vi "editDialog.vi"(0 "reference":refnum<class "StateNode.lvclass">, 1 "insidePackageNode":bool, 5 "error in (no error)":errorcluster) -> (14 "reference out":refnum<class "StateNode.lvclass">, 15 "changeConnection":T1, 16 "cancel":bool, 19 "error out":errorcluster)   [LabVIEW 2012, in "StateNode.lvclass"]
doc: "Edit Dialog"
uses:
  <resource>/Framework/Providers/Open_GDS/UML/StateNode_class/StateNode.lvclass
  <resource>/Framework/Providers/Open_GDS/UML/AbstractNode_class/private/NodeConnectionStatsType.ctl
  <resource>/Framework/Providers/Open_GDS/UML/ContextHelp/ContextHelp_HelpTexts.ctl
  <resource>/Framework/Providers/Open_GDS/UML/MultiLineString_class/MultiLineString.lvclass
  <resource>/Framework/Providers/Open_GDS/UML/AbstractNode_class/AbstractNode.lvclass
panel:
  in  "Action":string
  in  "OK Button":bool
  in  "Cancel Button":bool
  in  "Help":bool
  in  "State":string
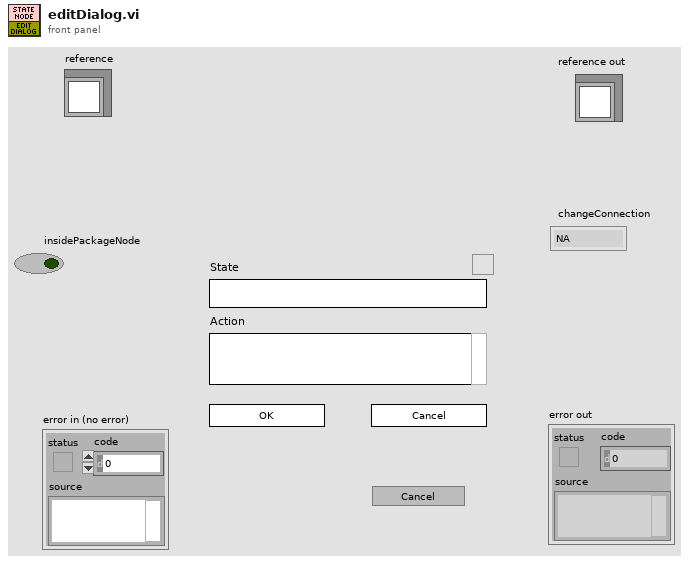
[diagram p1: front panel]
types:
  T1 = typedef "AbstractNode.lvclass/NodeConnectionStatsType.ctl" = enum16{"NA", "Connect", "DisConnect"}
  T2 = typedef "ContextHelp_HelpTexts.ctl" = enum16{"None(Hide)", "Default", "Help", "Welcome", "GettingStarted", "ClassDiagram_Help", "SequenceDiagram_Help", "UseCaseDiagram_Help", "BSelect", "BClass", "BInterface", "BPackage", "BNote", "BDependency", "BInheritance", "BInterfaceImplementation", "BAssociation", "BAggregation", "BCompAggregation", "BNoteConnector", "BObject", "BActionBar", "BCall", "BSystem", "BActor", "BUseCase", "BGeneralization", "BIncludes", "BExtends", "BUseCaseDiagramAssociation", "ClassRelationshipEdge editDialog_Bent Style", "ClassRelationshipEdge editDialog_RelationType", "ClassRelationshipEdge editDialog_Reverse association", "ClassRelationshipEdge editDialog_Start label", "ClassRelationshipEdge editDialog_Middle label", "ClassRelationshipEdge editDialog_End label", "UMLEditor reversedEngineering_Pathes", "ReversedEngineering StateReverseDialog_Help", "ReversedEngineering StateQueuedSettings_Help", "UMLEditor reversedEngineering_AddTopVIs", "UMLEditor reversedEngineering_AddClasses", "UMLEditor reversedEngineering_AddDirs", "UMLEditor reversedEngineering_Recursively", "UMLEditor reversedEngineering_Remove", "UMLEditor reversedEngineering_ClearList", "UMLEditor reversedEngineering_HideSubAss", "UMLEditor reversedEngineering_CreateTypes", "UMLEditor reversedEngineering_OnlyInheritance", "UMLEditor reversedEngineering_CreateApplication", "UMLEditor reversedEngineering_OK", "UMLEditor reversedEngineering_Cancel", "UMLEditor reversedEngineering_Help", "UMLEditor createWizardScriptFile_ScriptfilePath", "UMLEditor createWizardScriptFile_ClassPath", "UMLEditor createWizardScriptFile_Use", "UMLEditor createWizardScriptFile_PrivateDirName", "UMLEditor createWizardScriptFile_DirAppend", "UMLEditor createWizardScriptFile_Separator Character", "UMLEditor createWizardScriptFile_OK", "UMLEditor createWizardScriptFile_Cancel", "UMLEditor createWizardScriptFile_Help", "ClassNode editDialog_Class Name", "InterfaceNode editDialog_Class Name", "ClassNode editDialog_Attribute", "ClassNode editDialog_Methods", "InterfaceNode editDialog_Methods", "ClassNode editDialog_connection", "InterfaceNode editDialog_connection", "ClassNode editDialog_StereoType", "ClassNode editDialog_ShowAttrib", "ClassNode editDialog_ShowMethods", "ClassNode editDialog_ClassPath", "ClassNode editDialog_AddAttribute", "ClassNode editDialog_AddMethod", "InterfaceNode editDialog_AddMethod", "ClassNode AttributeGuide_AttributeName", "ClassNode AttributeGuide_Array?", "ClassNode AttributeGuide_Data Type", "ClassNode AttributeGuide_RefName", "ClassNode AttributeGuide_Preview", "ClassNode AttributeGuide_OK", "ClassNode AttributeGuide_Cancel", "ClassNode MethodGuide_Visibility", "ClassNode MethodGuide_Method Name", "ClassNode MethodGuide_Preview", "ClassNode MethodGuide_OK", "ClassNode MethodGuide_Cancel", "CallNode EditCallProperties_AllButtons", "ObjectNode EditObjectlProperties_AllButtons", "ActorNode EditActorProperties_AllButtons", "UseCaseRelationshipNode EditUseCaselProperties_AllButtons", "UseCaseNode EditUseCaselProperties_AllButtons", "SystemNode EditSystemProperties_AllButtons", "ReversedEngineering UpdateAttributes_AllButtons", "StateNode editDialog_AllButtons", "StateTransition editDialog_AllButtons", "ArrangeNodes Main_Picture", "ArrangeNodes Main_Zoom", "ArrangeNodes Main_Auto Zoom", "ArrangeNodes Main_shorten", "ArrangeNodes Main_Min Length", "ArrangeNodes Main_Max Length", "ArrangeNodes Main_increase", "ArrangeNodes Main_decrease", "ArrangeNodes Main_Shake", "ArrangeNodes Main", "BState", "BInitialState", "BFinalState", "BStateTransition", "StateDiagram_Help", "StateDiagram_PropertiesAllButtons", "ReversedEngineering StateReverseDialog_ClearStates", "ReversedEngineering StateReverseDialog_UseQueuedStateMachines", "ReversedEngineering StateReverseDialog_QueuedSettings", "ReversedEngineering StateReverseDialog_SearchForVIs", "ReversedEngineering StateReverseDialog_SearchCriteria", "OptionsDialog_ClassBasePath", "OptionsDialog_VIPath", "OptionsDialog_ApplicationPath", "OptionsDialog_WizDir", "OptionsDialog_IniFilePath", "OptionsDialog_DefineColors", "OptionsDialog_Help", "OptionsDialog_CreateTypes", "ClassRelationshipEdge editDialog_SplitWire"}
  T3 = typedef "StateNode.lvclass/ObjectAttributes.ctl" = cluster{"Base class":T4, "state":refnum<class "MultiLineString.lvclass">, "action":refnum<class "MultiLineString.lvclass">, "DEFAULT_WIDTH":i32, "DEFAULT_HEIGHT":i32}
  T4 = typedef "RectangularNode.lvclass/ObjectAttributes.ctl" = cluster{"Base class":T5, "bounds":T6}
  T5 = typedef "AbstractNode.lvclass/ObjectAttributes.ctl" = cluster{"parent":refnum<class "AbstractNode.lvclass">, "children":refnum<class "AbstractNode.lvclass">[], "Hidden":bool}
  T6 = typedef "Rectangle Rectangle2D.ctl" = cluster{"x":dbl, "y":dbl, "width":dbl, "height":dbl}
  T7 = typedef "ContextHelp_ShowType.ctl" = cluster{"Header":string, "Picture":picture, "Text":string}
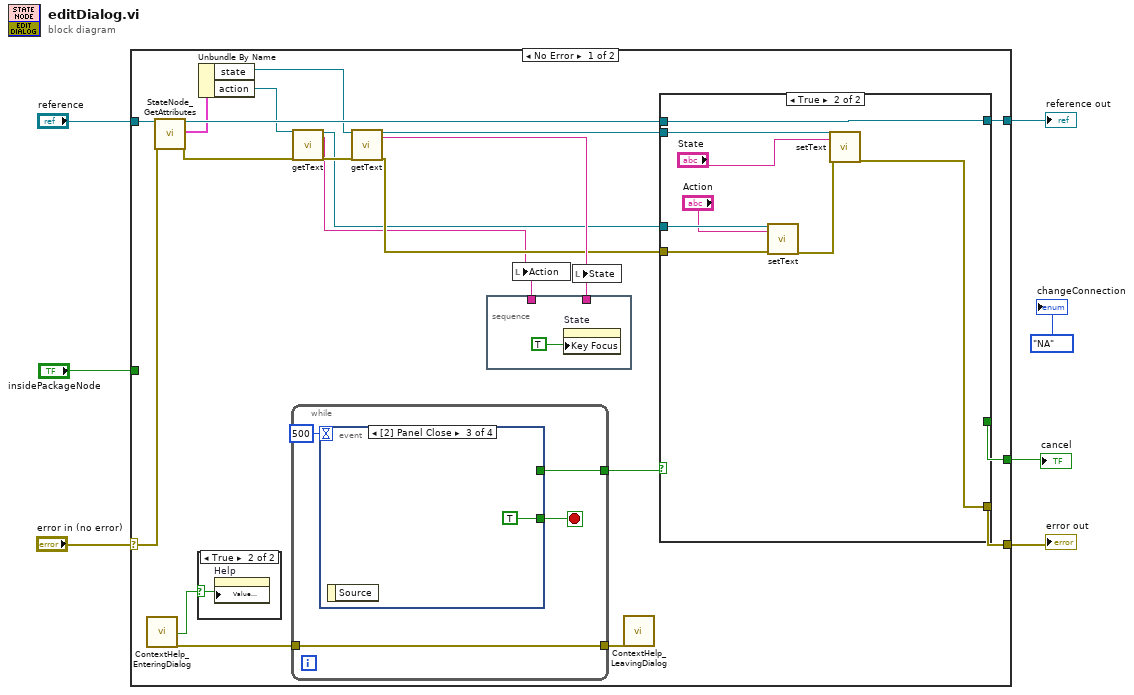
[diagram p0: block diagram]
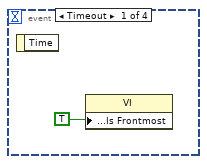
[diagram p3: hidden frame]
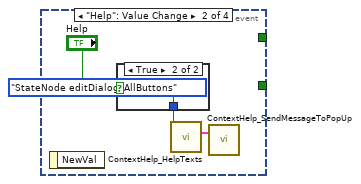
[diagram p4: hidden frame]
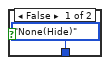
[diagram p5: hidden frame]
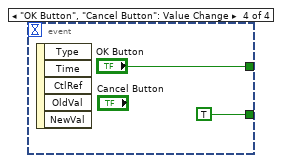
[diagram p6: hidden frame]
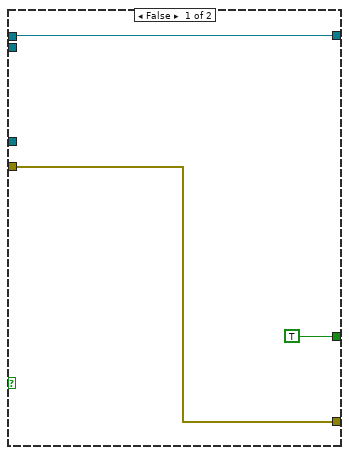
[diagram p7: hidden frame]
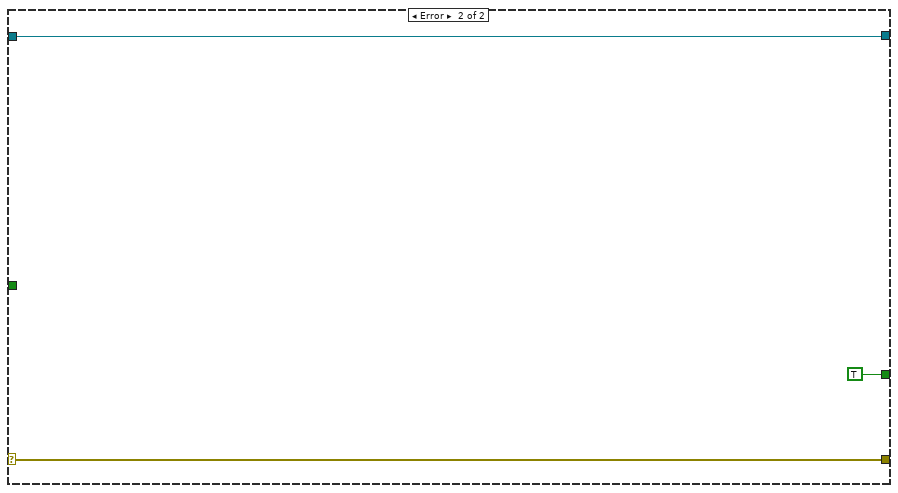
[diagram p8: hidden frame]
diagram:
  n1 = case shown="No Error" "error in (no error)" {
    selector: "error in (no error)" -> [w22 w54]
    tunnel: "reference" -> [w23 w55]
    tunnel: [w26 w54] -> w5
    tunnel: [w25 w55] -> w4
    tunnel: "insidePackageNode" -> [_ _]
    tunnel: [w16 TRUE ("Key Focus")] -> w2
    frame No Error {
      n2 = call <resource>:"ContextHelp_EnteringDialog.vi"() -> ("HelpStatus"=w11:bool, "error out"=w13:errorcluster)  [unwired: 3 in, 15 out]
      n3 = call <resource>:"StateNode_GetAttributes.vi"("reference in"=w23, "error in (no error)"=w22) -> ("reference out"=w24:refnum<class "StateNode.lvclass">, "Attributes"=w17:T3, "error out"=w21:errorcluster)  [unwired: 15 out]
      n4 = case shown="True" w11 {
        selector: w11 -> [_ w27]
        frame False {
        }
        frame True {
          n5 = property on="Help" class="Bool (strict)"("Value (Signaling)"=w27) -> ()  [unwired: 2 in, 2 out]
        }
      }
      n6 = Unbundle By Name(w17) -> ("state"=w18:refnum<class "MultiLineString.lvclass">, "action"=w10:refnum<class "MultiLineString.lvclass">)
      n7 = while {
        tunnel: [w31] -> w12
        tunnel: [w29] -> w14
        tunnel: w13 -> [w29]
        stop <- w30 stop-if-true
        n8 = event shown="[2] Panel Close" {
          selector: _ -> [_ _ _ _]
          dyn-events: _ -> [_ _ _ _]
          timeout: 500 -> [_ _ _ _]
          tunnel: [_ _ _ "OK Button"] -> w31
          tunnel: [_ _ TRUE TRUE] -> w30
          event Timeout {
            n9 = event-data() -> ()  [unwired: 2 out]
            n10 = property class="VI"("Front Panel Window:Is Frontmost"=TRUE) -> ()  [unwired: 2 in, 2 out]
          }
          event "Help": Value Change {
            n11 = event-data() -> ()  [unwired: 2 out]
            n12 = case shown="True" "Help" {
              tunnel: [ContextHelp_HelpTexts."None(Hide)" ("HelpText") ContextHelp_HelpTexts."StateNode editDialog_AllButtons" ("HelpText")] -> w34
              frame False {
              }
              frame True {
              }
            }
            n13 = call <resource>:"ContextHelp_HelpTexts.vi"("HelpText (enum or string)"=w34) -> ("HelpOut"=w35:T7)  [unwired: 18 out]
            n14 = call <resource>:"ContextHelp_SendMessageToPopUp.vi"("PopUpMessage"=w35) -> ()  [unwired: 2 in, 17 out]
          }
          event Panel Close {
            n15 = event-data() -> ()  [unwired: 2 out]
          }
          event "OK Button", "Cancel Button": Value Change {
            n16 = event-data() -> ()  [unwired: 6 out]
          }
        }
      }
      n17 = call-dynamic "getText.vi"("reference"=w10) -> ("reference out"=w8:refnum<class "MultiLineString.lvclass">, "text"=w9:string)  [unwired: 16 in, 1 out]
      n18 = call-dynamic "getText.vi"("reference"=w18, "error in (no error)"=w21) -> ("reference out"=w20:refnum<class "MultiLineString.lvclass">, "text"=w19:string, "error out"=w15:errorcluster)  [unwired: 15 in]
      n19 = stacked-sequence {
        tunnel: w19 -> [_]
        tunnel: w9 -> [_]
        frame #0 {
          n20 = property on="State" class="Str"("Key Focus"=TRUE) -> ()  [unwired: 2 in, 2 out]
        }
      }
      n21 = local write "Action"(w9) -> ()
      n22 = local write "State"(w19) -> ()
      n23 = call <resource>:"ContextHelp_LeavingDialog.vi"("error in (no error)"=w14) -> ()  [unwired: 2 in, 17 out]
      n24 = case shown="True" w12 {
        tunnel: [w42 w48] -> w26
        tunnel: [w43 w49] -> w25
        tunnel: w24 -> [w43 w49]
        tunnel: w20 -> [_ w51]
        tunnel: w15 -> [w42 w47]
        tunnel: [TRUE ("Key Focus") _] -> w16
        tunnel: w8 -> [_ w45]
        frame False {
        }
        frame True {
          n25 = call-dynamic "setText.vi"("reference"=w45, "text"="Action", "error in (no error)"=w47) -> ("error out"=w46:errorcluster)  [unwired: 15 in, 1 out]
          n26 = call-dynamic "setText.vi"("reference"=w51, "text"="State", "error in (no error)"=w46) -> ("error out"=w48:errorcluster)  [unwired: 15 in, 1 out]
        }
      }
    }
    frame Error {
    }
  }
  "reference out" <- w4
  "error out" <- w5
  "cancel" <- w2
  "changeConnection" <- NodeConnectionStatsType."NA" ("changeConnection")
